vi "Getting Started (TX on FPGA).vi"() -> ()   [LabVIEW 2017, in "My Network Host v1.lvlib"]
uses:
  My Network Host v1.lvlib
  <vilib>/userdefined/Silver/nirio_resource_slv.ctl
  <instrlib>/_niInstr/FIFO Register Bus/v1/Host/niInstr FIFO Register Bus v1 Host.lvclass
  C:/Program Files (x86)/National Instruments/LabVIEW 2017/instr.lib/_niInstr/Instruction Framework/v1/Host/Instruction Target/niInstr Instruction Target v1 Host.lvclass
  <instrlib>/_niInstr/Streaming/v1/Host/Public/Start Finite Stream.vi
  <instrlib>/_niInstr/Streaming/v1/Host/Public/Wait for Stream.vi
  <vilib>/FPGAPlugInAG/Dynamic/niLvFpga_Close_Dynamic.vi
  <vilib>/rvi/interface/nirviCloseFPGA/nirviCloseFPGA.xnode
  <instrlib>/_niInstr/Streaming/v1/Host/niInstr Streaming v1 Host.lvlib
  <instrlib>/_niInstr/Instruction Framework/v1/Host/Subsystem Map/niInstr Subsystem Map v1 Host.lvclass
  <instrlib>/_niInstr/Network/API/v1/Host/niInstr Network API Host v1.lvclass
panel:
  in  "UDP Destination Port":u16=35311
  out "CLIP state":T1
  out "error out":errorcluster
  in  "resource name":T2="RIO0"
  in  "MAC Source Address":u64=1108152157446 format="%012x"
  in  "MAC Destination Address":u64=281474976710655 format="%012x"
  in  "Local IP Address":string="169.254.122.138"
  in  "Dest IP Address":string="169.254.122.137"
  in  "TX Port":i32
  # "Example Setup\nNote: Compile the \"TenGbE_Project\" FPGA Target before running this VI. Error 7 \"File not found\" most likely means the bitfile has not been compiled yet.\n\n1. Choose the resource name for your device\n2. Plug a SFP+ Direct Attach cable to the TX Port and to the receiving Ethernet port\n3.  Choose a MAC Source Address for your port.  This needs to be a unique number on the network this is attached to.\n4. Optionally input the MAC Destination Address for the destination network card.  If this is not supplied, then using the default value of 0xFF... will broadcast the data to all reachable ports.\n5. Determine a unique Local IP Address for the FPGA.  This IP must be in the same subnet range as the target.\n6. Configure Dest IP Address to the IP address of the target Ethernet device.\nNote: in a host with more than one network card, this must be the IP address on the 10 GbE network card attached to the FPGA's network.\n7. Run a program on the target capable of capturing data on the specified UDP Destination Port\n8. Run this VI"
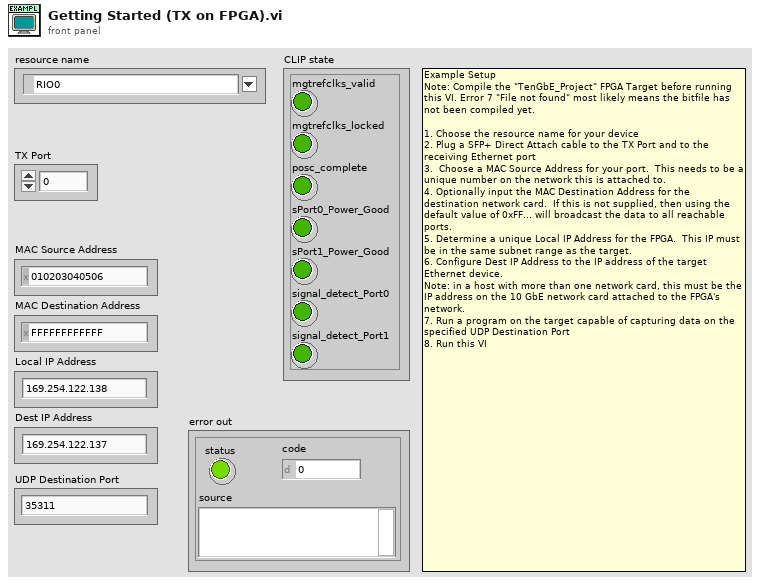
[diagram p1: front panel]
types:
  T1 = cluster{"mgtrefclks_valid":bool, "mgtrefclks_locked":bool, "posc_complete":bool, "sPort0_Power_Good":bool, "sPort1_Power_Good":bool, "signal_detect_Port0":bool, "signal_detect_Port1":bool}
  T2 = typedef "nirio_resource_slv.ctl" = tag
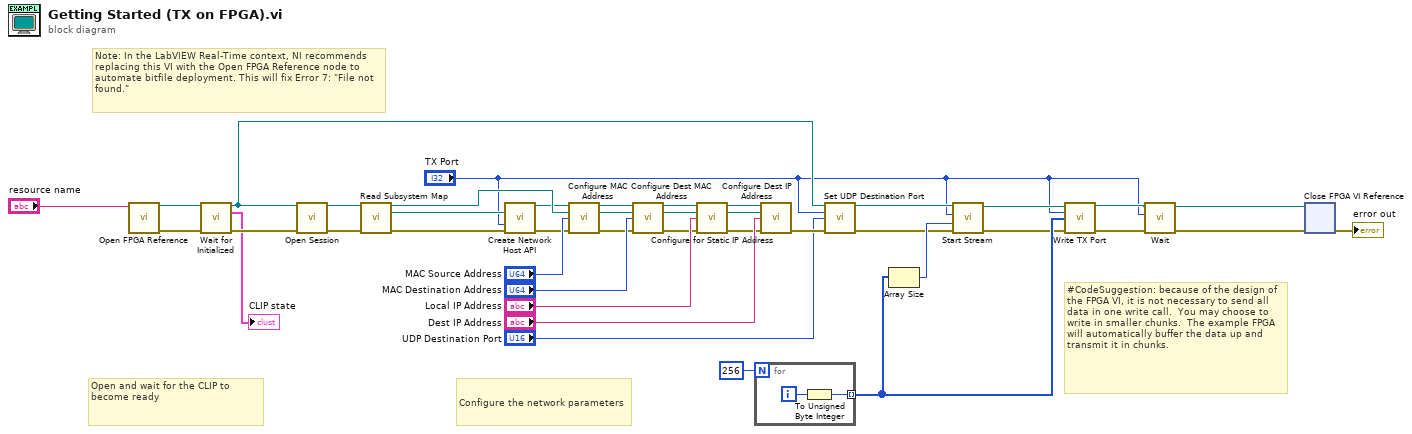
[diagram p0: block diagram]
diagram:
  # "Note: In the LabVIEW Real-Time context, NI recommends replacing this VI with the Open FPGA Reference node to automate bitfile deployment. This will fix Error 7: \"File not found.\""
  # "#CodeSuggestion: because of the design of the FPGA VI, it is not necessary to send all data in one write call.  You may choose to write in smaller chunks.  The example FPGA will automatically buffer the data up and transmit it in chunks."
  # "Configure the network parameters"
  # "Open and wait for the CLIP to become ready"
  n1 = call "Open FPGA Reference.vi"("resource name"="resource name") -> ("FPGA VI Reference Out"=w14:refnum<k20>, "error out"=w31:errorcluster)  [unwired: 13 in]
  n2 = call "Wait for Initialized.vi"("Refnum in"=w14, "error in (no error)"=w31) -> ("Refnum out"=w5:refnum<k20>, "CLIP state"=→"CLIP state":T1, "error out"=w30:errorcluster)  [unwired: 11 in]
  n3 = call <instrlib>:"Open Session.vi"("fpga ref"=w5, "error in"=w30) -> ("session out"=w41:refnum<class "niInstr FIFO Register Bus v1 Host.lvclass">, "error out"=w34:errorcluster)  [unwired: 12 in]
  n4 = call <instrlib>:"Read Subsystem Map.vi"("instruction target in"=w41, "error in"=w34) -> ("instruction target out"=w33:refnum<class "niInstr FIFO Register Bus v1 Host.lvclass">, "subsystem map"=w40:refnum<class "niInstr Subsystem Map v1 Host.lvclass">, "error out"=w35:errorcluster)  [unwired: 11 in]
  n5 = call <instrlib>:"Create Network Host API.vi"("subsystem map"=w40, "instance number"="TX Port", "error in (no error)"=w35) -> ("niInstr Network API Host v1 out"=w17:refnum<class "niInstr Network API Host v1.lvclass">, "error out"=w18:errorcluster)  [unwired: 11 in]
  n6 = call <instrlib>:"Configure MAC Address.vi"("niInstr Network API Host v1 in"=w17, "instruction target in"=w33, "Local MAC Address"="MAC Source Address", "error in (no error)"=w18) -> ("niInstr Network API Host v1 out"=w24:refnum<class "niInstr Network API Host v1.lvclass">, "instruction target out"=w25:refnum<class "niInstr FIFO Register Bus v1 Host.lvclass">, "error out"=w23:errorcluster)  [unwired: 9 in]
  n7 = call <instrlib>:"Configure Dest MAC Address.vi"("niInstr Network API Host v1 in"=w24, "instruction target in"=w25, "MAC Destination Address"="MAC Destination Address", "error in (no error)"=w23) -> ("niInstr Network API Host v1 out"=w26:refnum<class "niInstr Network API Host v1.lvclass">, "instruction target out"=w19:refnum<class "niInstr FIFO Register Bus v1 Host.lvclass">, "error out"=w20:errorcluster)  [unwired: 9 in]
  n8 = call <instrlib>:"Configure for Static IP Address.vi"("niInstr Network API Host v1 in"=w26, "instruction target in"=w19, "Local IP Address"="Local IP Address", "error in (no error)"=w20) -> ("niInstr Network API Host v1 out"=w27:refnum<class "niInstr Network API Host v1.lvclass">, "instruction target out"=w22:refnum<class "niInstr FIFO Register Bus v1 Host.lvclass">, "error out"=w21:errorcluster)  [unwired: 9 in]
  n9 = for {
    N: 256 -> [_]
    tunnel: [w42] -> w28 mode=indexing
    i -> [w43]
    n10 = To Unsigned Byte Integer(number=w43) -> (unsigned 8bit integer=w42:u8)
  }
  n11 = call <instrlib>:"Configure Dest IP Address.vi"("niInstr Network API Host v1 in"=w27, "instruction target in"=w22, "Dest IP Address"="Dest IP Address", "error in (no error)"=w21) -> ("error out"=w8:errorcluster)  [unwired: 9 in, 2 out]
  n12 = call "Set UDP Destination Port.vi"("Refnum in"=w5, "ethernet port"="TX Port", "UDP Destination Port"="UDP Destination Port", "error in (no error)"=w8) -> ("Refnum out"=w6:refnum<k20>, "error out"=w7:errorcluster)  [unwired: 10 in]
  n13 = Array Size(array=w28) -> (size(s)=w11:i32)
  n14 = call-poly <instrlib>:"Start Stream.vi"("error in (no error)"=w7, "num samples"=w11, "stream index"="TX Port", "refnum in"=w6) -> ("error out"=w13:errorcluster, "refnum out"=w12:refnum<k20>)  [unwired: 6 in]
  n15 = call "Write TX Port.vi"("Refnum in"=w12, "TX Port"="TX Port", "Data"=w28, "error in (no error)"=w13) -> ("Refnum out"=w10:refnum<k20>, "error out"=w9:errorcluster)  [unwired: 10 in]
  n16 = call-poly <instrlib>:"Wait.vi"("error in (no error)"=w9, "stream index"="TX Port", "refnum in"=w10) -> ("error out"=w15:errorcluster, "refnum out"=w16:refnum<k20>)  [unwired: 5 in, 2 out]
  n17 = xnode "Close FPGA VI Reference"("FPGA VI Reference In"=w16, "error in"=w15) -> ("error out"=→"error out":errorcluster)
